vi "Draw Arrow.vi"(8 "Draw Circle?":bool, 9 "Offset":cluster{"x":dbl, "y":dbl}, 10 "Theta":dbl, 11 "Radius":dbl) -> (2 "Endpoint":cluster{dbl, dbl}, 3 "Points":cluster{dbl[], dbl[]}[](array[cluster]))   [LabVIEW 2020]
uses:
  <vilib>/Analysis/coordinate.llb/2D Cartesian Coordinate Rotation (Array).vi
  <vilib>/Analysis/NI_AALPro.lvlib
panel:
  out "XY Graph":cluster{dbl[], dbl[]}[](graph)
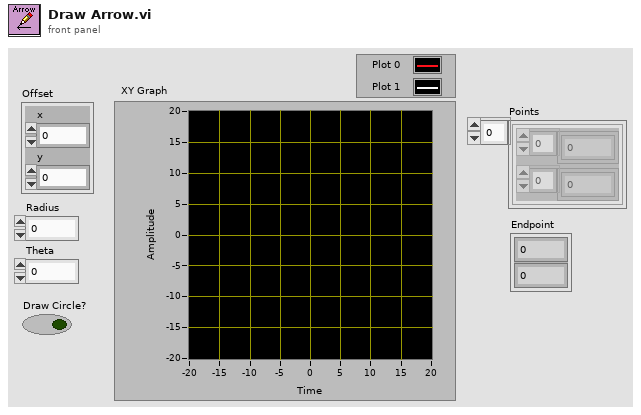
[diagram p1: front panel]
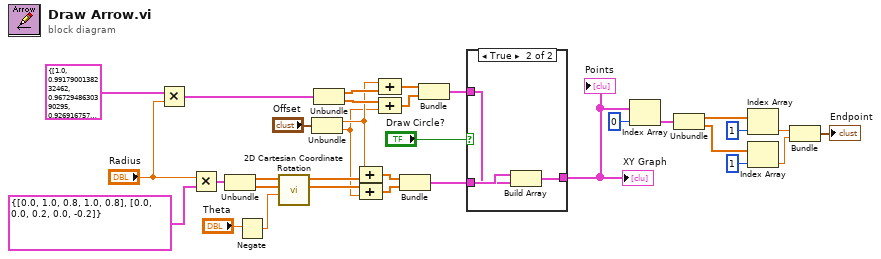
[diagram p0: block diagram]
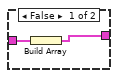
[diagram p2: hidden frame]
diagram:
  n1 = Multiply(x=cluster{dbl[], dbl[]} {[1.0, 0.9917900138232462, 0.9672948630390295, 0.9269167573460217, 0.8713187041233894, 0.8014136218679567, 0.7183493500977276, 0.6234898018587336, 0.5183925683105252, 0.404783343122394, 0.28452758663103267, 0.15959989503337932, 0.03205157757165533, -0.09602302590768154, -0.22252093395631434, -0.3453650544213075, -0.4625382902408351, -0.5721166601221694, -0.6723008902613166, -0.7614459583691342, -0.8380881048918404, -0.900968867902419, -0.9490557470106686, -0.9815591569910653, -0.9979453927503363, -0.9979453927503363, -0.9815591569910654, -0.9490557470106689, -0.9009688679024191, -0.8380881048918408, -0.7614459583691346, -0.672300890261317, -0.57211666012217, -0.4625382902408353, -0.34536505442130816, -0.2225209339563146, -0.09602302590768244, 0.03205157757165486, 0.1595998950333784, 0.284527586631032, 0.40478334312239295, 0.5183925683105245, 0.6234898018587334, 0.718349350097727, 0.8014136218679565, 0.871318704123389, 0.9269167573460216, 0.9672948630390291, 0.991790013823246, 1.0], [0.0, 0.127877161684506, 0.25365458390950735, 0.3752670048793741, 0.49071755200393785, 0.5981105304912159, 0.6956825506034864, 0.7818314824680298, 0.8551427630053461, 0.9144126230158124, 0.9586678530366606, 0.9871817834144502, 0.9994862162006879, 0.9953791129491982, 0.9749279121818236, 0.9384684220497604, 0.8865993063730001, 0.8201722545969561, 0.7402779970753157, 0.6482283953077888, 0.545534901210549, 0.43388373911755823, 0.3151082180236209, 0.19115862870137254, 0.06407021998071323, -0.06407021998071255, -0.19115862870137187, -0.3151082180236202, -0.433883739117558, -0.5455349012105485, -0.6482283953077882, -0.7402779970753153, -0.8201722545969556, -0.886599306373, -0.9384684220497602, -0.9749279121818236, -0.9953791129491981, -0.9994862162006879, -0.9871817834144503, -0.9586678530366608, -0.9144126230158128, -0.8551427630053464, -0.7818314824680299, -0.6956825506034869, -0.5981105304912162, -0.49071755200393863, -0.3752670048793746, -0.25365458390950835, -0.12787716168450664, -2.4492935982947064e-16]} ("output cluster"), y="Radius") -> (x*y=w20:cluster{dbl[], dbl[]})
  n2 = Multiply(x="Radius", y=cluster{dbl[], dbl[]} {[0.0, 1.0, 0.8, 1.0, 0.8], [0.0, 0.0, 0.2, 0.0, -0.2]}) -> (x*y=w32:cluster{dbl[], dbl[]})
  n3 = Unbundle(w32) -> (w31:dbl[], w30:dbl[])
  n4 = Negate(x="Theta") -> (-x=w23:dbl)
  n5 = call-poly <vilib>:"2D Cartesian Coordinate Rotation.vi"("theta"=w23, "Y"=w30, "X"=w31) -> ("Y Out"=w28:dbl[], "X Out"=w29:dbl[])  [unwired: 6 in, 1 out]
  n6 = Unbundle("Offset") -> ("x"=w17:dbl, "y"=w16:dbl)
  n7 = Unbundle(w20) -> (w19:dbl[], w18:dbl[])
  n8 = Compound Arithmetic op=ADD(w17, w29) -> (w26:dbl[])
  n9 = Compound Arithmetic op=ADD(w28, w16) -> (w25:dbl[])
  n10 = Compound Arithmetic op=ADD(w17, w19) -> (w14:dbl[])
  n11 = Compound Arithmetic op=ADD(w18, w16) -> (w13:dbl[])
  n12 = Bundle(w26, w25) -> (w12:cluster{dbl[], dbl[]})  [unwired: 1 in]
  n13 = Bundle(w14, w13) -> (w11:cluster{dbl[], dbl[]})  [unwired: 1 in]
  n14 = case shown="True" "Draw Circle?" {
    tunnel: w12 -> [w35 w38]
    tunnel: w11 -> [_ w37]
    tunnel: [w34 w36] -> w10
    frame False {
      n15 = Build Array(w35) -> (w34:cluster{dbl[], dbl[]}[])
    }
    frame True {
      n16 = Build Array(w38, w37) -> (w36:cluster{dbl[], dbl[]}[])
    }
  }
  "XY Graph" <- w10
  "Points" <- w10
  n17 = Index Array(array=w10, index=0) -> (element=w8:cluster{dbl[], dbl[]})
  n18 = Unbundle(w8) -> (w7:dbl[], w6:dbl[])
  n19 = Index Array(array=w7, index=1) -> (element=w3:dbl)
  n20 = Index Array(array=w6, index=1) -> (element=w2:dbl)
  n21 = Bundle(w3, w2) -> (→"Endpoint":cluster{dbl, dbl})  [unwired: 1 in]
